vi "SCM10_IO_Multi.vi"(4 "ERR IN":errorcluster={"status"=FALSE, "code"=-1073807343, "source"="Property Node (arg 2) in SCM10_IO_Multi.vi->SCM10_GetData_Multi.vi->VISAREADtest.vi"}, 5 "QUERY":string="RELST? 1", 6 "Delay (ms, Serial Only)":u32=100, 7 "I/O IN":T1={"I/O Select (Serial: 0)"=enum."Serial", "VISA"="ASRL0::INSTR", "IP Address"="192.168.111.127", "Baud Rate"=enum."115200", "COM"=1}) -> (0 "ERR OUT":errorcluster, 1 "RESPONSE":string="RELST 1,1\r", 2 "FAULT?":bool, 3 "I/O OUT":T1={"I/O Select (Serial: 0)"=enum."Serial", "VISA"="ASRL1::INSTR", "IP Address"="192.168.111.127", "Baud Rate"=enum."115200", "COM"=1})   [LabVIEW 2016]
uses:
  Instance           4 22Saved   SCM10_IO_Multi .vi
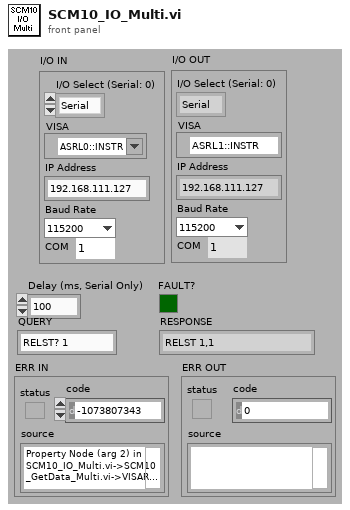
[diagram p1: front panel]
types:
  T1 = cluster{"I/O Select (Serial: 0)":enum16{"Serial", "TCP"}, "VISA":refnum<visa-resource-name>, "IP Address":string, "Baud Rate":enum16{"9600", "19200", "57600", "115200"}, "COM":i32}
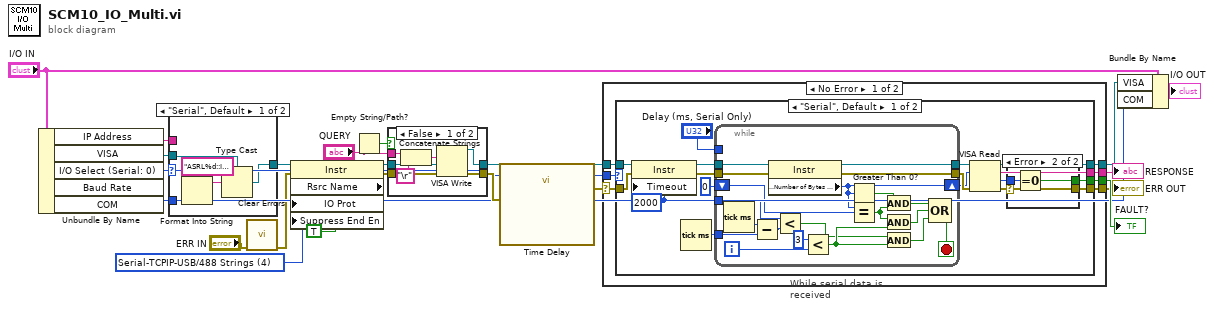
[diagram p0: block diagram]
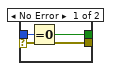
[diagram p2: hidden frame]
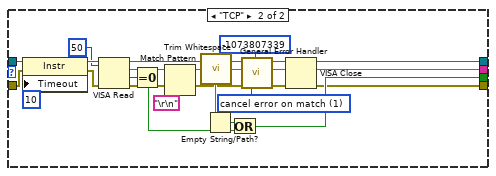
[diagram p3: hidden frame]
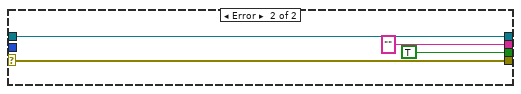
[diagram p4: hidden frame]
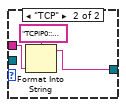
[diagram p5: hidden frame]
diagram:
  w14 = u16 4 items=["Normal"=1, "VXI/FDC"=2, "GPIB/HS488"=3, "Serial-TCPIP-USB/488 Strings"=4, "USBTMC/Vendor-Specific"=5] ("Message Based Settings:IO Protocol")
  n1 = Unbundle By Name("I/O IN") -> ("IP Address"=w7:string, "VISA"=w8:refnum<visa-resource-name>, "I/O Select (Serial: 0)"=w6:enum16{"Serial", "TCP"}, "COM"=w4:i32)  [unwired: 1 out]
  n2 = case shown="\"Serial\", Default" w6 {
    tunnel: w8 -> [w24 _]
    tunnel: w7 -> [_ w29]
    tunnel: [w23 w28] -> w5
    tunnel: w4 -> [w27 _]
    frame "Serial", Default {
      n3 = Format Into String(format string="ASRL%d::INSTR", w27) -> (resulting string=w25:string)  [unwired: 2 in, 1 out]
      n4 = Type Cast(type=w24, x=w25) -> (*(type *) &x=w23:refnum<visa-resource-name>)
    }
    frame "TCP" {
      n5 = Format Into String(format string="TCPIP0::%s::9760::SOCKET", w29) -> (resulting string=w28:string)  [unwired: 2 in, 1 out]
    }
  }
  n6 = call <vilib>:"Clear Errors.vi"("error in (no error)"="ERR IN") -> ("error out"=w2:errorcluster)  [unwired: 5 in, 1 out]
  n7 = property class="Instr" props=["Rsrc Name", "IO Prot", "Suppress End En"](reference=w5, error in=w2, "IO Prot"=w14, "Suppress End En"=TRUE ("Message Based Settings:Suppress End Enable")) -> (reference out=w18:refnum<visa-resource-name>, error out=w17:errorcluster)  [unwired: 1 out]
  n8 = Empty String/Path?(string/path="QUERY") -> (empty?=w15:bool)
  n9 = case shown="False" w15 {
    tunnel: [w37 w39] -> w16
    tunnel: w18 -> [w36 w39]
    tunnel: w17 -> [w35 w38]
    tunnel: [w34 w38] -> w9
    tunnel: "QUERY" -> [w31 _]
    frame False {
      n10 = Concatenate Strings(w31, "\r") -> (w33:string)
      n11 = VISA Write(VISA resource name=w36, write buffer=w33, error in (no error)=w35) -> (VISA resource name out=w37:refnum<visa-resource-name>, error out=w34:errorcluster)  [unwired: 1 out]
    }
    frame True {
    }
  }
  n12 = call "Time Delay"("error in (no error)"=w9) -> ("error out"=w3:errorcluster)  [unwired: 10 in]
  n13 = case shown="No Error" w3 {
    selector: w3 -> [w40 w111]
    tunnel: w16 -> [w46 w113]
    tunnel: [w45 "" ("trimmed string")] -> w12
    tunnel: [w44 TRUE] -> w11
    tunnel: [w43 w113] -> w10
    tunnel: [w42 w111] -> w1
    tunnel: w6 -> [w41 _]
    frame No Error {
      n14 = case shown="\"Serial\", Default" w41 {
        tunnel: [w49 w90] -> w42
        tunnel: [w53 w92] -> w43
        tunnel: w46 -> [w60 w109]
        tunnel: w40 -> [w59 w108]
        tunnel: [w50 w96] -> w44
        tunnel: [w48 w99] -> w45
        frame "Serial", Default {
          w47 = u32 2000 ("General Settings:Timeout Value")
          n15 = property class="Instr"(reference=w60, error in=w59, "Timeout"=w47) -> (reference out=w57:refnum<visa-resource-name>, error out=w58:errorcluster)
          n16 = Tick Count (ms)() -> (millisecond timer value=w62:u32)
          n17 = while "While serial data is received" {
            tunnel: w57 -> [w89]
            tunnel: w58 -> [w70]
            tunnel: w62 -> [w88]
            tunnel: w47 -> [w85]
            shift-right: [w79] -> w54
            shift-left: u32 0 ("Serial Settings:Number of Bytes at Serial Port") -> [w84]
            tunnel: "Delay (ms, Serial Only)" -> [_]
            tunnel: [w83] -> w55
            tunnel: [w82] -> w56
            i -> [w80]
            stop <- w78 stop-if-true
            n18 = Tick Count (ms)() -> (millisecond timer value=w87:u32)
            n19 = Subtract(x=w87, y=w88) -> (x-y=w86:u32)
            n20 = property class="Instr"(reference=w89, error in=w70) -> (reference out=w82:refnum<visa-resource-name>, error out=w83:errorcluster, "Serial Settings:Number of Bytes at Serial Port"=w79:u32)
            n21 = Less?(x=w85, y=w86) -> (x < y?=w74:bool)
            n22 = Less?(x=3 ("y"), y=w80) -> (x < y?=w75:bool)
            n23 = Greater Than 0?(x=w79) -> (x > 0?=w77:bool)
            n24 = Equal?(x=w79, y=w84) -> (x = y?=w76:bool)
            n25 = And(x=w77, y=w76) -> (x .and. y?=w71:bool)
            n26 = And(x=w76, y=w75) -> (x .and. y?=w72:bool)
            n27 = And(x=w74, y=w75) -> (x .and. y?=w73:bool)
            n28 = Compound Arithmetic op=OR(w71, w72, w73) -> (w78:bool)
          }
          n29 = VISA Read(VISA resource name=w56, byte count=w54, error in (no error)=w55) -> (VISA resource name out=w53:refnum<visa-resource-name>, read buffer=w48:string, return count=w51:u32, error out=w52:errorcluster)
          n30 = case shown="Error" w52 {
            selector: w52 -> [w66 w69]
            tunnel: [w66 w69] -> w49
            tunnel: [w65 w68] -> w50
            tunnel: w51 -> [w64 w67]
            frame No Error {
              n31 = Equal To 0?(x=w64) -> (x = 0?=w65:bool)
            }
            frame Error {
              n32 = Equal To 0?(x=w67) -> (x = 0?=w68:bool)
            }
          }
        }
        frame "TCP" {
          w93 = 1 items=["no exception", "cancel error on match", "set error on match"] ("[exception action] (none:0)")
          n33 = property class="Instr"(reference=w109, error in=w108, "Timeout"=u32 10 ("General Settings:Timeout Value")) -> (reference out=w106:refnum<visa-resource-name>, error out=w105:errorcluster)
          n34 = VISA Read(VISA resource name=w106, byte count=u32 50, error in (no error)=w105) -> (VISA resource name out=w92:refnum<visa-resource-name>, read buffer=w102:string, return count=w100:u32, error out=w95:errorcluster)
          n35 = Equal To 0?(x=w100) -> (x = 0?=w97:bool)
          n36 = Match Pattern(string=w102, regular expression="\r\n") -> (before substring=w101:string)  [unwired: 1 in, 3 out]
          n37 = call <vilib>:"Trim Whitespace.vi"("string"=w101) -> ("trimmed string"=w99:string)  [unwired: 1 in]
          n38 = Empty String/Path?(string/path=w99) -> (empty?=w98:bool)
          n39 = Or(x=w98, y=w97) -> (x .or. y?=w96:bool)
          n40 = call <vilib>:"General Error Handler.vi"("error in (no error)"=w95, "[exception action] (none:0)"=w93, "[exception code]"=-1073807339) -> ("error out"=w91:errorcluster)  [unwired: 8 in, 4 out]
          n41 = VISA Close(VISA resource name=w92, error in (no error)=w91) -> (error out=w90:errorcluster)
        }
      }
    }
    frame Error {
    }
  }
  "ERR OUT" <- w1
  "RESPONSE" <- w12
  "FAULT?" <- w11
  n42 = Bundle By Name(cluster="I/O IN", "VISA"=w10, "COM"=w4) -> (→"I/O OUT":T1)
